vi "Init Database.vi"(8 "error in (no error)":errorcluster, 9 "Database":string, 10 "Resource":string, 11 "Database in":refnum<class "SQLite.lvclass">) -> (0 "error out":errorcluster, 3 "Database out":refnum<class "SQLite.lvclass">)   [LabVIEW 2020, in "Conditum SQLite.lvlib" / "SQLite.lvclass"]
uses:
  SQLite.lvclass
  <vilib>/drjdpowell/SQLite Library/SQL Connection/Connection.lvclass
  <vilib>/drjdpowell/SQLite Library/SQL Connection/Open (string).vi
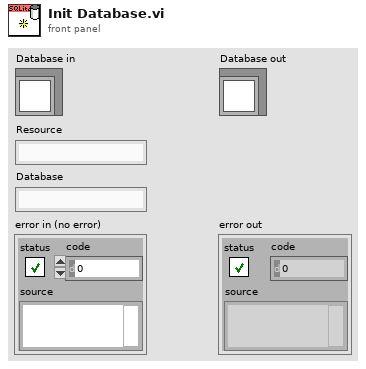
[diagram p1: front panel]
types:
  T1 = enum16{"New or existing", "Existing", "Read only"}
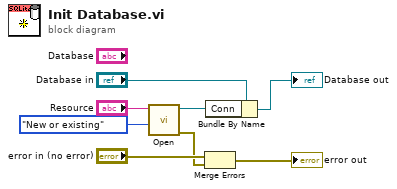
[diagram p0: block diagram]
diagram:
  n1 = call-poly <vilib>:"Open.vi"("File Option"=T1."New or existing", "db file"="Resource") -> ("error out"=w1:errorcluster, "SQLite Connection"=w3:refnum<class "Connection.lvclass">)  [unwired: 8 in]
  n2 = Merge Errors("error in (no error)", w1) -> (→"error out":errorcluster)
  n3 = Bundle By Name(cluster="Database in", "Conn"=w3) -> (→"Database out":refnum<class "SQLite.lvclass">)
